vi "ATF-Pump NS Connect.vi"(8 "error in (no error)":errorcluster, 11 "Pump Ip Address":string) -> (0 "error out 2":errorcluster, 2 "writer endpoint":refnum<k21>, 3 "reader endpoint":refnum<k21>)   [LabVIEW 2022 SP3]
uses:
  Controls/SeCrTs-NS Data type.ctl
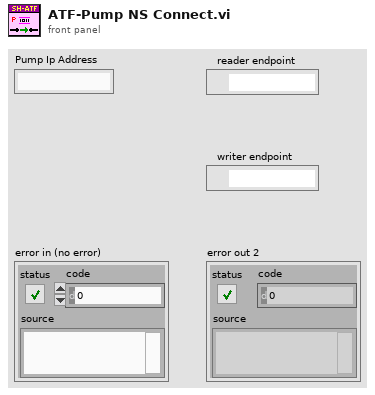
[diagram p1: front panel]
types:
  T1 = typedef "SeCrTs-NS Data type.ctl" = cluster{"DI_Data":digitalwaveform[], "Drive_A_C":waveform(dbl)[], "Drive_A_D":waveform(dbl)[], "Drive_L_C":waveform(dbl)[], "Drive_L_D":waveform(dbl)[], "Loop Status":bool[], "CDT":dbl, "RT Error":cluster{"Error Code":string, "Error Source":string}, "DO":waveform(dbl)[], "SEQ Monitor":string[], "Device List":string}
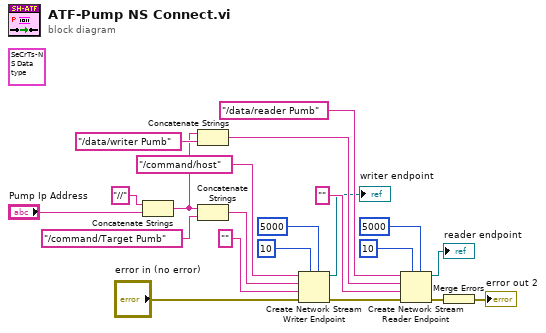
[diagram p0: block diagram]
diagram:
  (unwired) T1 {"DI_Data"=[], "Drive_A_C"=[], "Drive_A_D"=[], "Drive_L_C"=[], "Drive_L_D"=[], "Loop Status"=[], "CDT"=0.0, "RT Error"={"Error Code"="", "Error Source"=""}, "DO"=[], "SEQ Monitor"=[], "Device List"=""}
  n1 = Concatenate Strings("//" ("reader url"), "Pump Ip Address") -> (w9:string)
  n2 = Concatenate Strings(w9, "/data/writer Pumb" ("reader url")) -> (w14:string)
  n3 = Concatenate Strings(w9, "/command/Target Pumb" ("reader url")) -> (w13:string)
  n4 = Create Network Stream Writer Endpoint(5:5000 ("timeout in ms (-1)"), 7:10 ("timeout in ms (-1)"), 8:"error in (no error)", 9:"" ("concatenated string"), 10:w13, 11:"/command/host" ("writer name")) -> (0:w16:errorcluster, 3:→"writer endpoint":refnum<k21>)  [unwired: 1 in]
  n5 = Create Network Stream Reader Endpoint(5:5000 ("timeout in ms (-1)"), 7:10 ("reader buffer size"), 8:w16, 9:"" ("concatenated string"), 10:w14, 11:"/data/reader Pumb" ("writer name")) -> (0:w20:errorcluster, 3:→"reader endpoint":refnum<k21>)  [unwired: 1 in]
  n6 = Merge Errors(w20) -> (→"error out 2":errorcluster)
